vi "Setup.vi"(7 "Sender":refnum<class "Sender.lvclass">, 11 "Setup in":refnum<class "Setup.lvclass">) -> (3 "Setup out":refnum<class "Setup.lvclass">)   [LabVIEW 2021, in "jettl.lvlib" / "Setup Msg.lvlib" / "Setup.lvclass"]
uses:
  Setup.lvclass
  Sender/Sender/Sender.lvclass
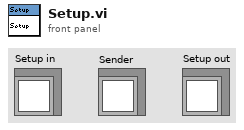
[diagram p1: front panel]
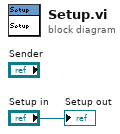
[diagram p0: block diagram]
diagram:
  "Setup out" <- "Setup in"
